vi "Parse.vi"(8 "error in (no error)":errorcluster, 11 "Transform.Matrix in":refnum<class "Transform.Matrix.lvclass">) -> (0 "error out":errorcluster, 3 "Transform.Matrix out":refnum<class "Transform.Matrix.lvclass">)   [LabVIEW 2019, in "Transform.Matrix.lvclass"]
uses:
  Transform.Matrix.lvclass
  C:/Users/Albro/Documents/GitHub/AFM-Lithography/lvsrc/Classes/Parse/Transform/Transform.lvclass
  <vilib>/Utility/error.llb/whitespace.ctl
  Transform/Transform.lvclass/Transform.ctl
  Transform/Transform.lvclass
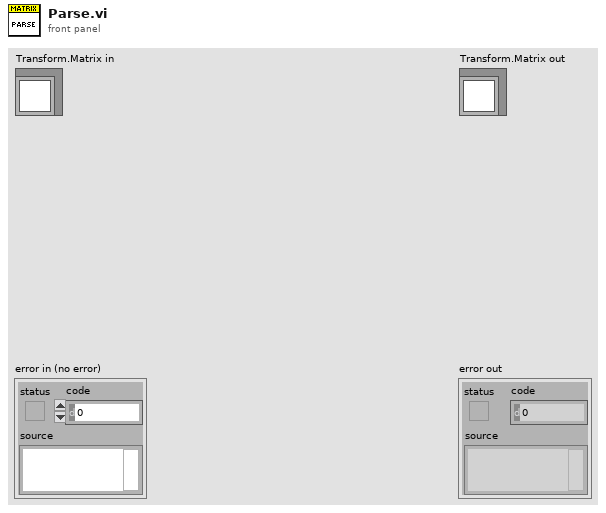
[diagram p1: front panel]
types:
  T1 = typedef "whitespace.ctl" = u16
  T2 = typedef "NI_Matrix.lvlib/RealMatrix.ctl" = dbl[][]
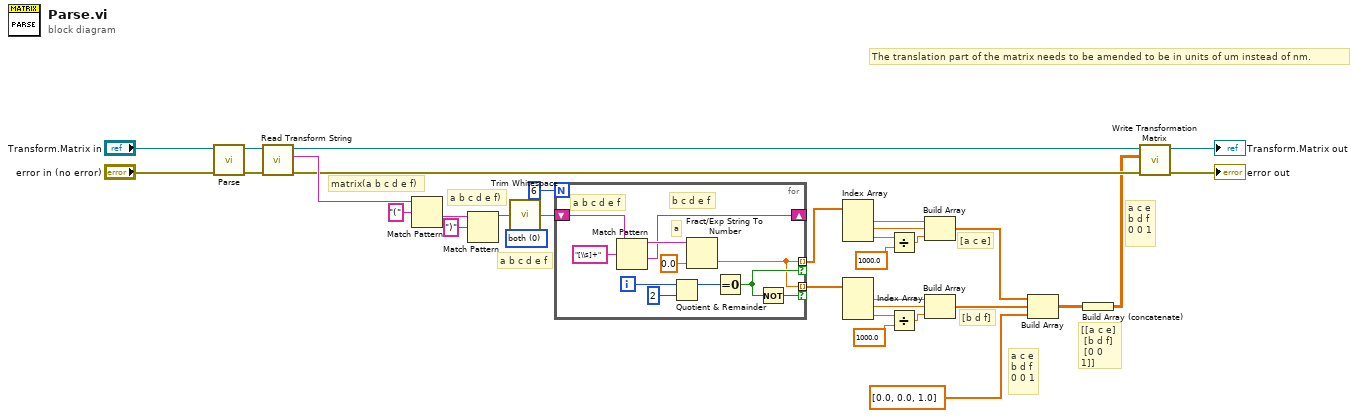
[diagram p0: block diagram]
diagram:
  w24 = T1 0 items=["both", "start of string", "end of string"] ("location (both)")
  # "The translation part of the matrix needs to be amended to be in units of um instead of nm."
  # "[b d f]"
  # "a c e \nb d f \n0 0 1"
  # "a c e \nb d f \n0 0 1"
  # "[[a c e] \n [b d f] \n [0 0 1]]"
  # "[a c e]"
  # "a b c d e f"
  # "a b c d e f)"
  # "matrix(a b c d e f)"
  n1 = call-parent "Parse.vi"("error in (no error)"="error in (no error)", "Transform in"="Transform.Matrix in") -> ("error out"=w25:errorcluster, "Transform out"=w32:refnum<class "Transform.Matrix.lvclass">)  [unwired: 8 in]
  n2 = call "Read Transform String.vi"("error in (no error)"=w25, "Transform in"=w32) -> ("error out"=w20:errorcluster, "Transform String"=w31:string, "Transform out"=w22:refnum<class "Transform.Matrix.lvclass">)  [unwired: 7 in]
  n3 = Match Pattern(string=w31, regular expression="(") -> (after substring=w23:string)  [unwired: 1 in, 3 out]
  n4 = Match Pattern(string=w23, regular expression=")") -> (before substring=w28:string)  [unwired: 1 in, 3 out]
  n5 = call <vilib>:"Trim Whitespace.vi"("string"=w28, "location (both)"=w24) -> ("trimmed string"=w27:string)
  n6 = for {
    N: 6 -> [_]
    shift-right: [w40] -> _
    shift-left: w27 -> [w43]
    tunnel: [w34] -> w10 mode=indexing if=w35
    tunnel: [w34] -> w3 mode=indexing if=w36
    i -> [w39]
    # "a"
    # "b c d e f"
    # "a b c d e f"
    n7 = Match Pattern(string=w43, regular expression="[\\s]+") -> (before substring=w42:string, after substring=w40:string)  [unwired: 1 in, 2 out]
    n8 = Quotient & Remainder(x=w39, y=2) -> (x-y*floor(x/y)=w37:i32)  [unwired: 1 out]
    n9 = Fract/Exp String To Number(string=w42, default (0 dbl)=0.0 ("default (0 DBL)")) -> (number=w34:dbl)  [unwired: 2 in, 1 out]
    n10 = Equal To 0?(x=w37) -> (x = 0?=w35:bool)
    n11 = Not(x=w35) -> (.not. x?=w36:bool)
  }
  n12 = Index Array(array=w10) -> (element #1=w13:dbl, element #2=w14:dbl, element #3=w15:dbl)  [unwired: 3 in]
  n13 = Index Array(array=w3) -> (element #1=w6:dbl, element #2=w5:dbl, element #3=w4:dbl)  [unwired: 3 in]
  n14 = Divide(x=w15, y=1000.0) -> (x/y=w12:dbl)
  n15 = Divide(x=w4, y=1000.0) -> (x/y=w7:dbl)
  n16 = Build Array(w13, w14, w12) -> (w9:dbl[])
  n17 = Build Array(w6, w5, w7) -> (w2:dbl[])
  n18 = Build Array(w9, w2, dbl[] [0.0, 0.0, 1.0] ("element")) -> (w17:dbl[][])
  n19 = Build Array (concatenate)(w17) -> (w16:T2)
  n20 = call "Write Transformation Matrix.vi"("error in (no error)"=w20, "Real Matrix"=w16, "Transform in"=w22) -> ("error out"=→"error out":errorcluster, "Transform out"=→"Transform.Matrix out":refnum<class "Transform.Matrix.lvclass">)  [unwired: 7 in]
